vi "Write Quantum Desing Configuration.vi"(8 "error in (no error)":errorcluster, 10 "Quantum Desing Configuration":T1={"Address"="127.0.0.1", "Instrument type"=0, "Remote"=FALSE, "Temperature"=FALSE, "Field"=FALSE} {"Instrument type" items=["PPMS", "VersaLab", "DynaCool", "SVSM"]}, 11 "Quantum Design Driver in":refnum<class "Quantum Design Driver.lvclass">) -> (0 "error out":errorcluster, 3 "Quantum Design Driver out":refnum<class "Quantum Design Driver.lvclass">)   [LabVIEW 2018, in "Quantum Design Driver.lvclass"]
uses:
  Quantum Design Driver.lvclass
  C:/github/NHMFL_Core/Libraries/Instruments/Instrument Driver/Instrument Driver.lvclass
  Quantum Desing Configuration.ctl
  Instrument Driver/Write User configuration.vi
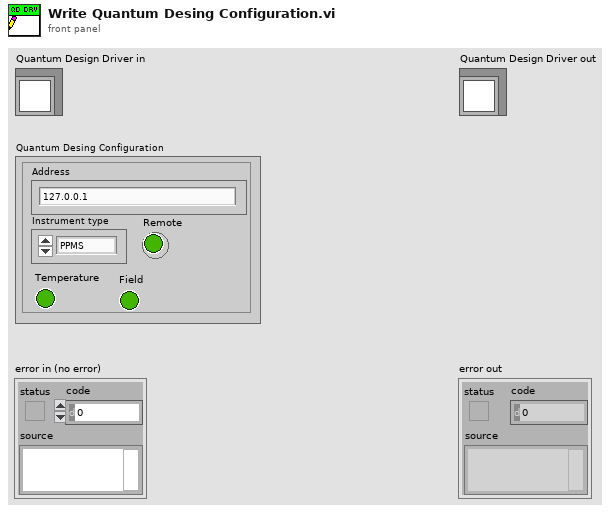
[diagram p1: front panel]
types:
  T1 = typedef "Quantum Desing Configuration.ctl" = cluster{"Address":string, "Instrument type":u16, "Remote":bool, "Temperature":bool, "Field":bool}
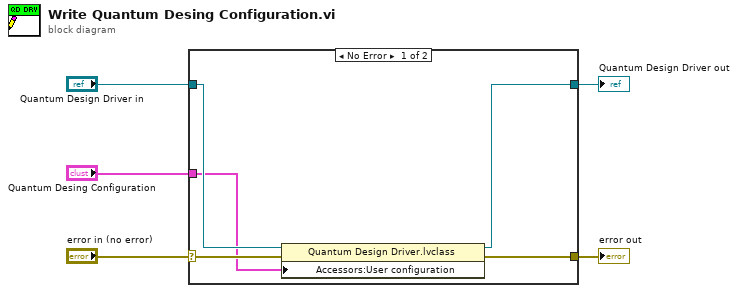
[diagram p0: block diagram]
diagram:
  n1 = case shown="No Error" "error in (no error)" {
    selector: "error in (no error)" -> [w10 w11]
    tunnel: [w9 w11] -> w4
    tunnel: [w7 w12] -> w2
    tunnel: "Quantum Design Driver in" -> [w8 w12]
    tunnel: "Quantum Desing Configuration" -> [w6 _]
    frame No Error {
      n2 = property class="Quantum Design Driver.lvclass"(reference=w8, error in=w10, "Accessors:User configuration"=w6) -> (reference out=w7:refnum<class "Quantum Design Driver.lvclass">, error out=w9:errorcluster)
    }
    frame Error {
    }
  }
  "error out" <- w4
  "Quantum Design Driver out" <- w2
